vi "Projet programmation, partie Labview.vi"() -> ()   [LabVIEW 2013]
uses:
  <vilib>/Analysis/Matrix/Datatypes/RealMatrix.ctl
  <vilib>/Analysis/Matrix/NI_Matrix.lvlib
panel:
  out "error out":errorcluster
  out "computed command line":string="computed command line"
  out "OS Name":string="Mac"
  out "standard matlab error":string
  out "standard matlab output":string
  out "output cluster":cluster{string, string}
  in  "Representation des points non-filtre":string(combo)
  in  "Style du signal non-filtre":string(combo)
  in  "Couleur du signal non-filtre":string(combo)
  out "Spreadsheet string":string
  out "appended array":T1
  in  "Representation des points filtres":string(combo)
  in  "Style du signal filtre":string(combo)
  in  "Couleur du signal fitre":string(combo)
  out "Signal final":dbl[](array[numeric])
  out "Signal filtre":dbl[](array[numeric])
  out "Waveform Graph":dbl[](graph)
  out "Genere_cpp Return code":i32
  out "Chemin de F_periode.txt":path
  out "file or folder exists?":bool
  out "Standard Genere_cpp error":string
  out "Standard Genere_cpp output":string
  out "VI name":string
  out "Chemin de l'executable":path
  out "EntrŽe dans CMD":string
  in  "Forme du signal":enum32{"sinus", "carrŽ"}(radio)
  out "Array":dbl[](array[numeric])
  out "String du F_periode.txt":string
  in  "Numero echant":i32=8
  in  "Filtre":bool
  in  "Nombre periodes":dbl
  in  "Nombre Points":dbl=8.0 min=8.0 max=256.0
  in  "Bruit":dbl(knob) min=0.0 max=10.0 scale=0.0..10.0 scale format="%#_4g"
  in  "Offset":dbl(knob) min=-5.0 max=5.0 step=0.001 scale=-5.0..5.0 scale format="%#_4g"
  in  "Amplitude":dbl(knob) min=0.0 max=10.0 step=0.001 scale=0.0..10.0 scale format="%#.4g"
  # "Control Panel"
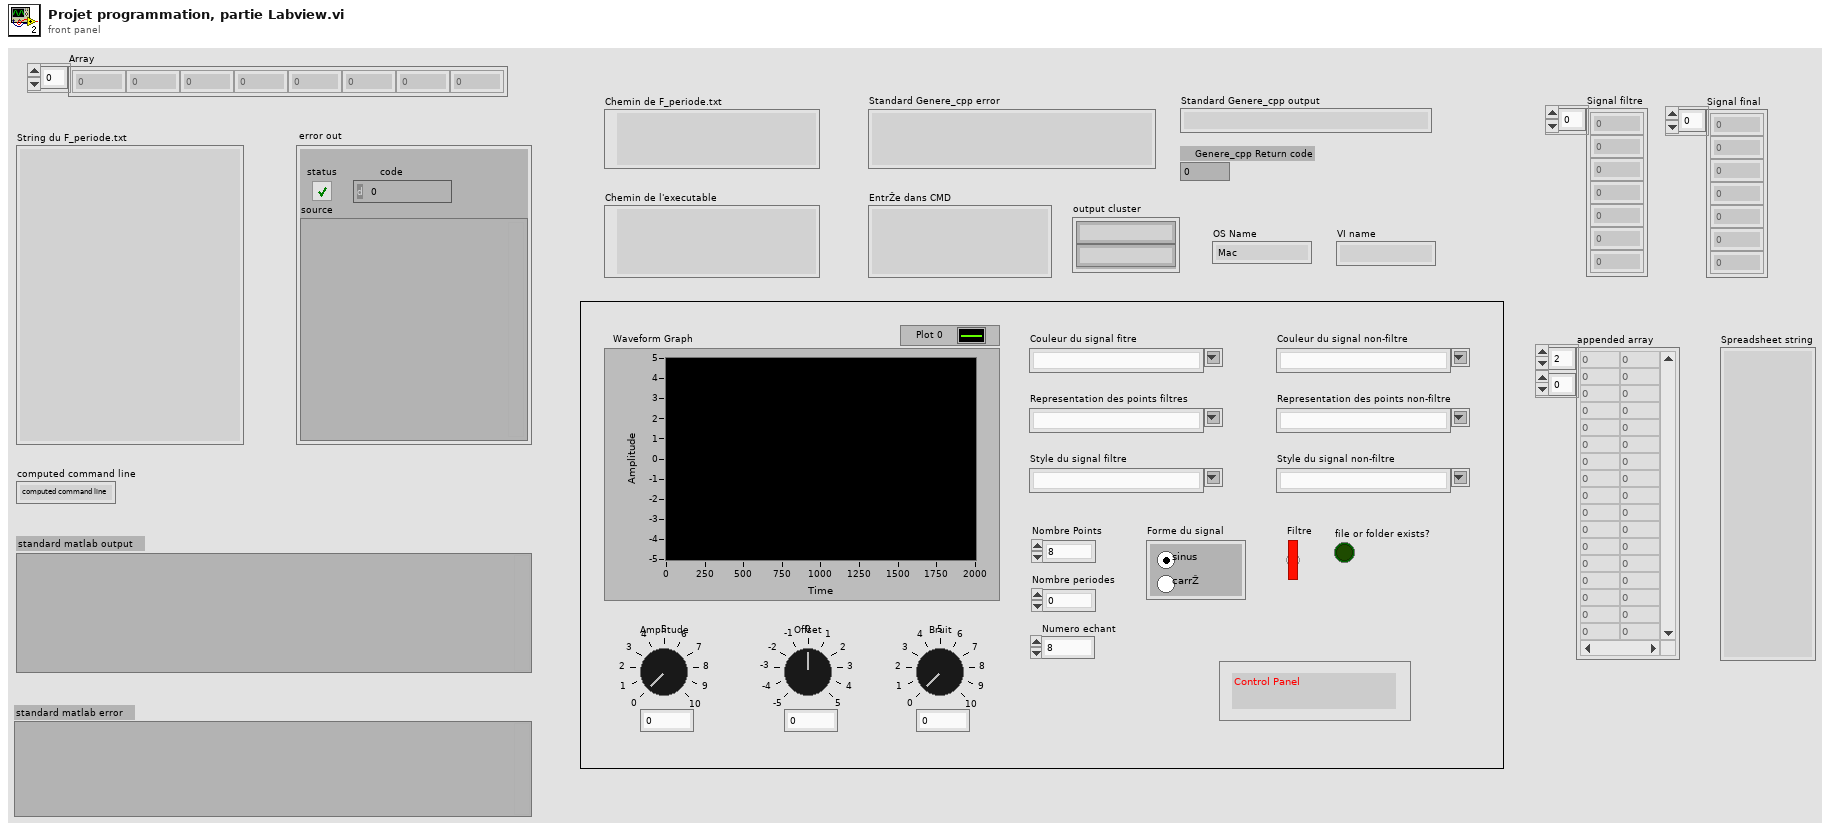
[diagram p1: front panel]
types:
  T1 = typedef "NI_Matrix.lvlib/RealMatrix.ctl" = dbl[][]
  T2 = enum16{"open", "replace", "create", "open or create", "replace or create", "replace or create with confirmation"}
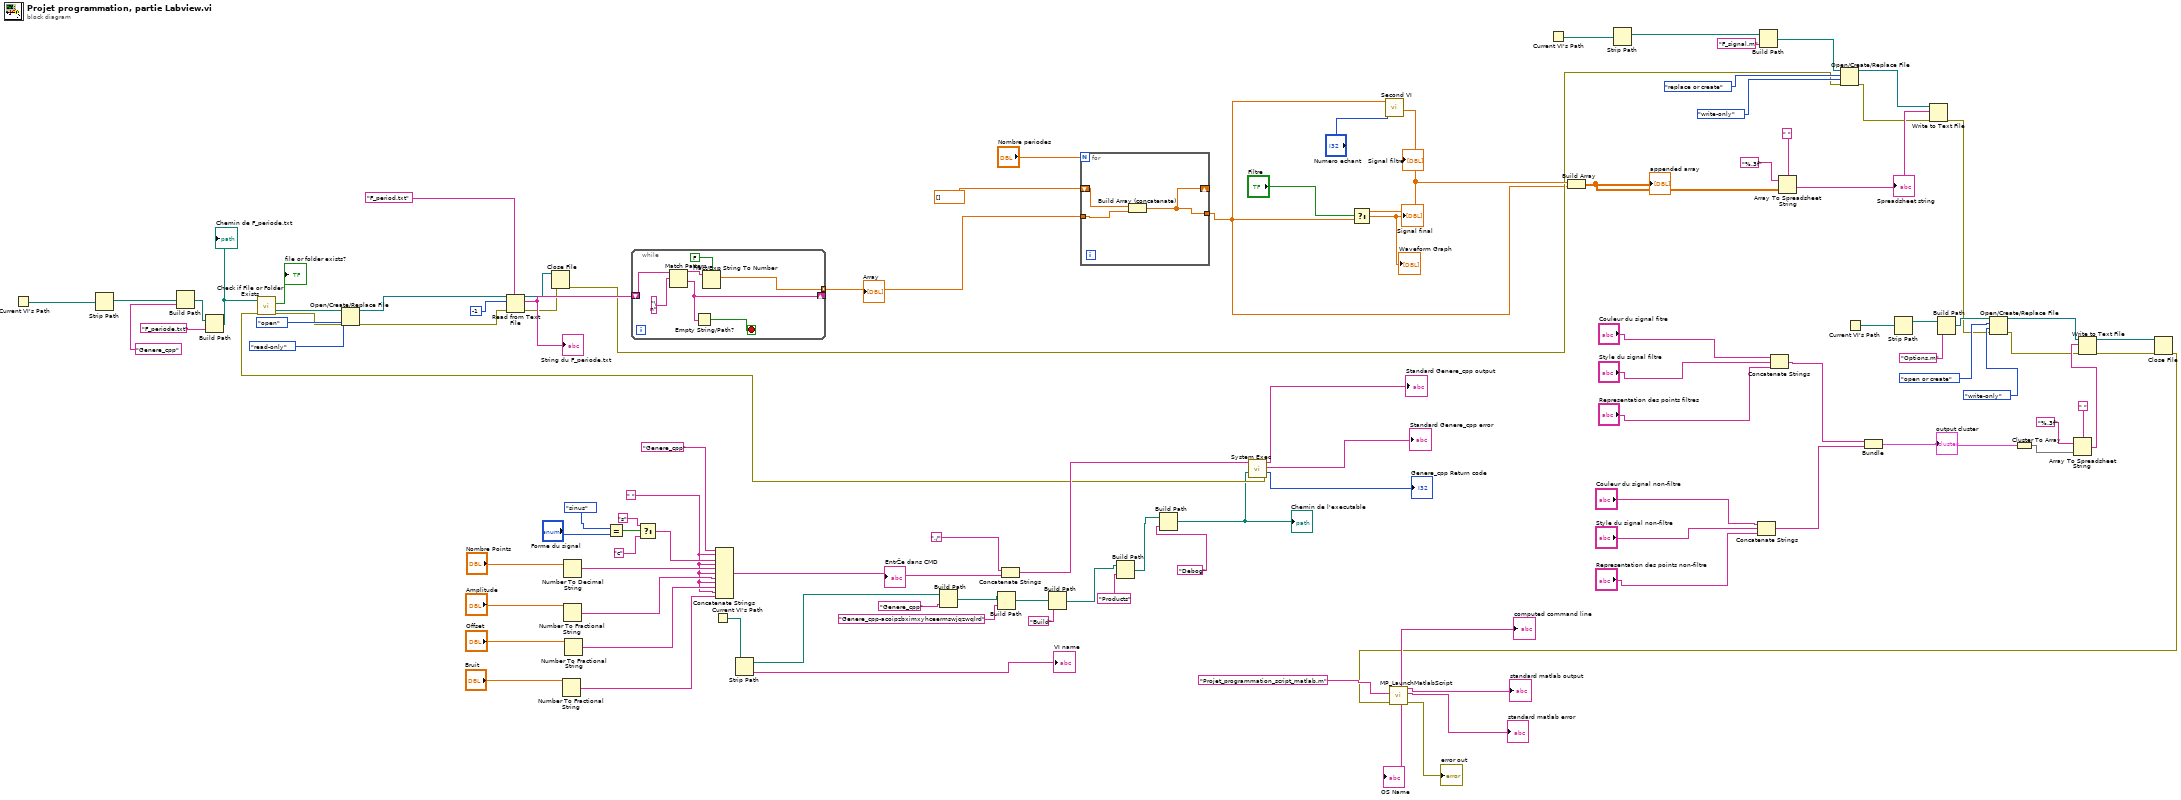
[diagram p0: block diagram]
diagram:
  w85 = " "
  n1 = Current VI's Path() -> (path=w75:path)
  n2 = Strip Path(path=w75) -> (stripped path=w74:path)  [unwired: 1 out]
  n3 = Build Path(base path=w74, name or relative path="Genere_cpp") -> (appended path=w70:path)
  n4 = Build Path(base path=w70, name or relative path="F_periode.txt") -> (appended path=w69:path)
  "Chemin de F_periode.txt" <- w69
  n5 = Number To Fractional String(number="Bruit") -> (F-format string=w86:string)  [unwired: 3 in]
  n6 = Number To Fractional String(number="Amplitude") -> (F-format string=w88:string)  [unwired: 3 in]
  n7 = Number To Decimal String(number="Nombre Points") -> (decimal integer string=w89:string)  [unwired: 1 in]
  n8 = Number To Fractional String(number="Offset") -> (F-format string=w87:string)  [unwired: 3 in]
  n9 = Equal?(x=enum32{"sinus", "carrŽ"}."sinus" ("Forme"), y="Forme du signal") -> (x = y?=w97:bool)
  n10 = Select(t="s", s=w97, f="c") -> (s? t:f=w90:string)
  n11 = Current VI's Path() -> (path=w84:path)
  n12 = Concatenate Strings("Genere_cpp", w85, w90, w85, w89, w85, w88, w85, w87, w85, w86) -> (w81:string)
  "EntrŽe dans CMD" <- w81
  n13 = Strip Path(path=w84) -> (stripped path=w72:path, name=→"VI name":string)
  n14 = Build Path(base path=w72, name or relative path="Genere_cpp") -> (appended path=w28:path)
  n15 = Build Path(base path=w28, name or relative path="Genere_cpp-acoipzbximxyhceermswjqzwqlrd") -> (appended path=w27:path)
  n16 = Concatenate Strings("./", w81) -> (w80:string)
  n17 = Build Path(base path=w27, name or relative path="Build") -> (appended path=w26:path)
  n18 = Build Path(base path=w26, name or relative path="Products") -> (appended path=w22:path)
  n19 = Build Path(base path=w22, name or relative path="Debog") -> (appended path=w1:path)
  "Chemin de l'executable" <- w1
  n20 = call <vilib>:"System Exec.vi"("working directory"=w1, "command line"=w80) -> ("error out"=w13:errorcluster, "return code"=→"Genere_cpp Return code":i32, "standard error"=→"Standard Genere_cpp error":string, "standard output"=→"Standard Genere_cpp output":string)  [unwired: 6 in]
  n21 = call <vilib>:"Check if File or Folder Exists.vi"("error in (no error)"=w13, "path"=w69) -> ("error out"=w12:errorcluster, "file or folder exists?"=→"file or folder exists?":bool, "dup path"=w106:path)  [unwired: 7 in]
  n22 = Open/Create/Replace File(file path (use dialog)=w106, error in=w12, operation (0:open)=T2."open", access (0:read/write)=enum16{"read/write", "read-only", "write-only"}."read-only") -> (refnum out=w105:refnum<file>, error out=w11:errorcluster)  [unwired: 2 in, 1 out]
  n23 = Read from Text File(prompt (Open existing file)="F_period.txt", file (use dialog)=w105, count=-1, error in=w11) -> (refnum out=w20:refnum<file>, text=w100:string, error out=w10:errorcluster)  [unwired: 1 out]
  "String du F_periode.txt" <- w100
  n24 = Close File(refnum=w20, error in=w10) -> (error out=w9:errorcluster)  [unwired: 1 out]
  n25 = while {
    shift-right: [w113] -> _
    shift-left: w100 -> [w110]
    tunnel: [w109] -> w64 mode=indexing
    stop <- w112 stop-if-true
    n26 = Match Pattern(string=w110, regular expression="\n") -> (before substring=w111:string, after substring=w113:string)  [unwired: 1 in, 2 out]
    n27 = Empty String/Path?(string/path=w113) -> (empty?=w112:bool)
    n28 = Fract/Exp String To Number(use system decimal point (T)=FALSE, string=w111) -> (number=w109:dbl)  [unwired: 2 in, 1 out]
  }
  "Array" <- w64
  n29 = for {
    N: "Nombre periodes" -> [_]
    tunnel: w64 -> [w116]
    shift-right: [w114] -> _
    shift-left: dbl[] [] ("Array 2") -> [w115]
    tunnel: [w114] -> w2
    n30 = Build Array (concatenate)(w115, w116) -> (w114:dbl[])
  }
  n31 = call "Second VI.vi"("Numero echant"="Numero echant", "Array"=w2) -> ("Array 2"=w61:dbl[])  [unwired: 9 in]
  "Signal filtre" <- w61
  n32 = Select(t=w61, s="Filtre", f=w2) -> (s? t:f=→"Waveform Graph" →"Signal final":dbl[])
  n33 = Current VI's Path() -> (path=w57:path)
  n34 = Build Array(w61, w2) -> (w8:T1)
  "appended array" <- w8
  n35 = Strip Path(path=w57) -> (stripped path=w56:path)  [unwired: 1 out]
  n36 = Concatenate Strings("Couleur du signal non-filtre", "Style du signal non-filtre", "Representation des points non-filtre") -> (w44:string)
  n37 = Build Path(base path=w56, name or relative path="F_signal.m") -> (appended path=w55:path)
  n38 = Concatenate Strings("Couleur du signal fitre", "Style du signal filtre", "Representation des points filtres") -> (w45:string)
  n39 = Array To Spreadsheet String(delimiter (Tab)=" ", array=w8, 3:"%.3f" ("format string")) -> (spreadsheet string=w52:string)
  "Spreadsheet string" <- w52
  n40 = Open/Create/Replace File(file path (use dialog)=w55, error in=w9, operation (0:open)=T2."replace or create", access (0:read/write)=enum16{"read/write", "read-only", "write-only"}."write-only") -> (refnum out=w53:refnum<file>, error out=w7:errorcluster)  [unwired: 2 in, 1 out]
  n41 = Current VI's Path() -> (path=w35:path)
  n42 = Bundle(w45, w44) -> (w43:cluster{string, string})  [unwired: 1 in]
  "output cluster" <- w43
  n43 = Strip Path(path=w35) -> (stripped path=w34:path)  [unwired: 1 out]
  n44 = Write to Text File(file (use dialog)=w53, text=w52, error in=w7) -> (error out=w6:errorcluster)  [unwired: 1 in, 2 out]
  n45 = Build Path(base path=w34, name or relative path="Options.m") -> (appended path=w37:path)
  n46 = Open/Create/Replace File(file path (use dialog)=w37, error in=w6, operation (0:open)=T2."open or create", access (0:read/write)=enum16{"read/write", "read-only", "write-only"}."write-only") -> (refnum out=w38:refnum<file>, error out=w5:errorcluster)  [unwired: 2 in, 1 out]
  n47 = Cluster To Array(cluster=w43) -> (array=w42:string[])
  n48 = Array To Spreadsheet String(delimiter (Tab)=" ", array=w42, 3:"%.3f" ("format string")) -> (spreadsheet string=w39:string)
  n49 = Write to Text File(file (use dialog)=w38, text=w39, error in=w5) -> (refnum out=w29:refnum<file>, error out=w4:errorcluster)  [unwired: 1 in, 1 out]
  n50 = Close File(refnum=w29, error in=w4) -> (error out=w3:errorcluster)  [unwired: 1 out]
  n51 = call "MP_LaunchMatlabScript.vi"("error in (no error)"=w3, "Projet_programmation_script_matlab.m"="Projet_programmation_script_matlab.m") -> ("error out"=→"error out":errorcluster, "standard error"=→"standard matlab error":string, "standard output"=→"standard matlab output":string, "OS Name"=→"OS Name":string, "computed command line"=→"computed command line":string)  [unwired: 5 in]
